vi "ext_cmd_sensitivity.vi"(11 "which clamp":enum16{"VClamp", "IClamp"}(ring)) -> (3 "division factor":dbl)   [LabVIEW 2019]
panel:
  # "EXTERNAL CMD SENSITIVITY"
  # "USAGE: INPUT / DIVISION FACTOR = OUTPUT"
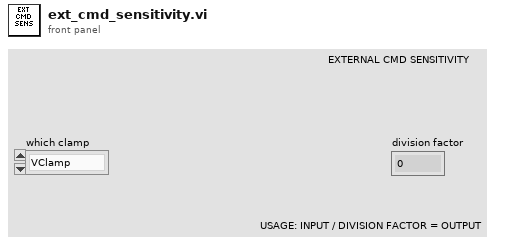
[diagram p1: front panel]
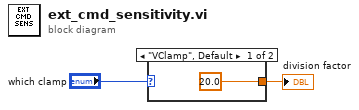
[diagram p0: block diagram]
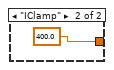
[diagram p2: hidden frame]
diagram:
  n1 = case shown="\"VClamp\", Default" "which clamp" {
    tunnel: [20.0 400.0] -> w1
    frame "VClamp", Default {
    }
    frame "IClamp" {
    }
  }
  "division factor" <- w1
